vi "WaitForElevatorCommand.vi"(10 "Numeric":dbl) -> ()   [LabVIEW 2014]
doc: "Wait for PIDInPositionDwell to be true.\n\nThe numeric is used to ensure scripts run in order. The input is NOT USED."
uses:
  Robot Global Data.vi
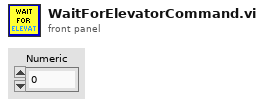
[diagram p1: front panel]
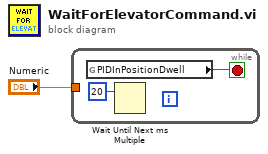
[diagram p0: block diagram]
diagram:
  n1 = while {
    tunnel: "Numeric" -> [_]
    stop <- w3 stop-if-true
    n2 = global read "Robot Global Data.vi" "PIDInPositionDwell"() -> (w3:bool)
    n3 = Wait Until Next ms Multiple(millisecond multiple=u32 20) -> ()  [unwired: 1 out]
  }
